vi "Initalize.vi"(3 "error in (no error)":errorcluster, 5 "Instruments in":refnum<class "Instruments.lvclass">) -> (0 "error out":errorcluster, 1 "Instruments out":refnum<class "Instruments.lvclass">)   [LabVIEW 2012, in "Instruments.lvclass"]
uses:
  Instruments.lvclass
  Instruments.lvclass/Instruments.ctl
panel:
  out "Ophir Board":string
  out "Debug Index":i32
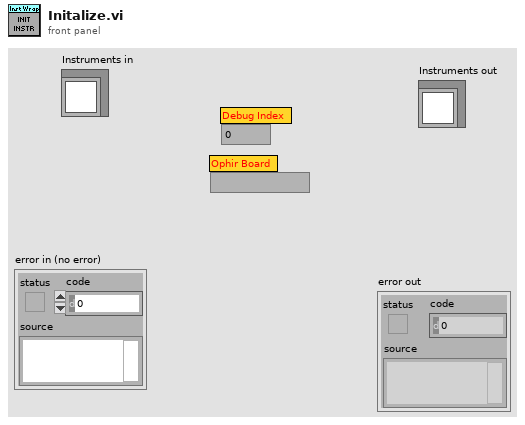
[diagram p1: front panel]
types:
  T1 = typedef "USB4000_Data.ctl" = cluster{"Wrapper Out":u32, "Number of Spectrometers":i32, "Wavelength":dbl[], "EL Spectrum":dbl[], "Int Time (usec)":i32, bool, "Background":dbl[]}
  T2 = typedef "OphirRef.ctl" = cluster{"OphirComRef":refnum<k7>, "deviceHandle":i32, "Channel":i32, "SerialNumber":string, "Background Wl":dbl, "Background":dbl, "CalWl":dbl}
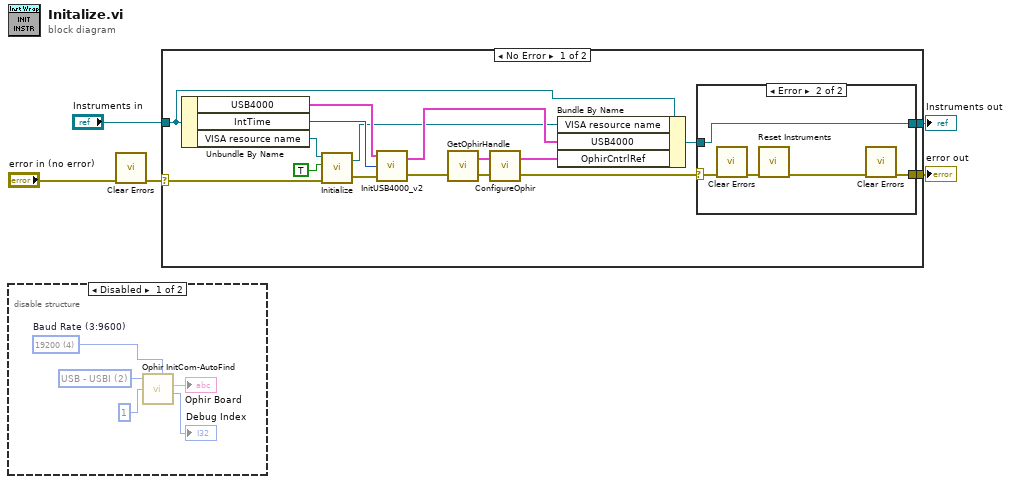
[diagram p0: block diagram]
diagram:
  n1 = disable-structure shown="Disabled" {
    frame Disabled {
      w8 = i16 4 items=["300", "1200", "4800", "9600", "19200", "38400"]  # Baud Rate (3:9600)
      w6 = i16 2 items=["USB - Nova2", "USB - Vega", "USB - USBI", "RS232", "GPIB"] ("communication")
      n2 = call "Ophir InitCom-AutoFind.vi"("Baud Rate (3:9600)"=w8, "communication"=w6, "Port Number (default 2)"=i16 1) -> ("Ophir Board"=→"Ophir Board":string, "Debug Index"=→"Debug Index":i32)  [unwired: 1 in, 2 out]
    }
    frame Enabled {
    }
  }
  n3 = call <vilib>:"Clear Errors.vi"("error in (no error)"="error in (no error)") -> ("error out"=w1:errorcluster)  [unwired: 6 in]
  n4 = case shown="No Error" w1 {
    selector: w1 -> [w25 w36]
    tunnel: [w15 w36] -> w5
    tunnel: [w13 w35] -> w3
    tunnel: "Instruments in" -> [w20 w35]
    frame No Error {
      n5 = Unbundle By Name(w20) -> ("USB4000"=w18:T1, "IntTime"=w19:i32, "VISA resource name"=w27:refnum<visa-resource-name>)
      n6 = call "Initialize.vi"("error in (no error)"=w25, "Reset (True)"=TRUE, "KE_In"=w27) -> ("error out"=w24:errorcluster, "KE_Out"=w17:refnum<visa-resource-name>)  [unwired: 1 in]
      n7 = call "InitUSB4000_v2.vi"("error in (no error)"=w24, "Int Time (usec)"=w19, "USB4000 In"=w18) -> ("error out"=w22:errorcluster, "USB4000 Out"=w23:T1)
      n8 = call "GetOphirHandle.vi"("error in (no error)"=w22) -> ("error out"=w11:errorcluster, "OphirRef Out"=w12:T2)  [unwired: 1 in]
      n9 = call "ConfigureOphir.vi"("error in (no error)"=w11, "OphirRef In"=w12) -> ("error out"=w16:errorcluster, "OphirRef Out"=w21:T2)
      n10 = Bundle By Name(cluster=w20, "VISA resource name"=w17, "USB4000"=w23, "OphirCntrlRef"=w21) -> (w14:refnum<class "Instruments.lvclass">)
      n11 = case shown="Error" w16 {
        selector: w16 -> [w29 w30]
        tunnel: [w29 w31] -> w15
        tunnel: w14 -> [w28 w32]
        tunnel: [w28 w32] -> w13
        frame No Error {
        }
        frame Error {
          n12 = call <vilib>:"Clear Errors.vi"("error in (no error)"=w30) -> ("error out"=w34:errorcluster)  [unwired: 6 in]
          n13 = call "Reset Instruments"("error in (no error)"=w34) -> ("error out"=w33:errorcluster)  [unwired: 9 in, 1 out]
          n14 = call <vilib>:"Clear Errors.vi"("error in (no error)"=w33) -> ("error out"=w31:errorcluster)  [unwired: 6 in]
        }
      }
    }
    frame Error {
    }
  }
  "error out" <- w5
  "Instruments out" <- w3
